vi "liberaToCmd.vi"(5 "set Time":string, 6 "loops":i32=1, 7 "acquire time":u32, 8 "samples":u32=1, 9 "triggered":bool, 10 "decimated":bool, 11 "cmd":T1(ring)=enum."acquireDD") -> (0 "jsonargs":string, 3 "cmd":string)   [LabVIEW 2010]
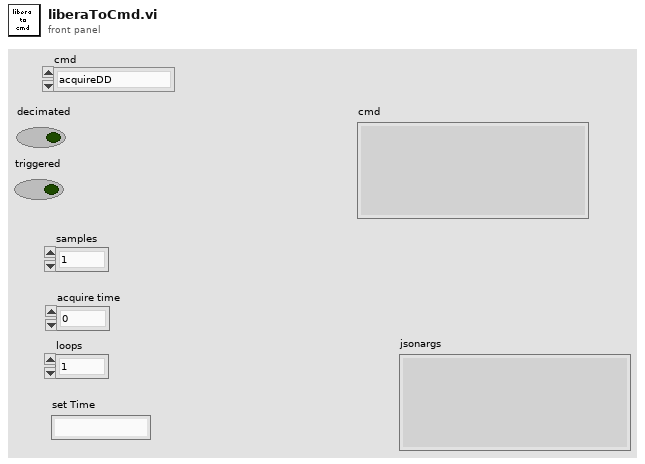
[diagram p1: front panel]
types:
  T1 = enum16{"stopAcquire", "setTime", "acquireAVG", "acquireADCSP", "acquireADCCW", "acquireStream", "acquireDD"}
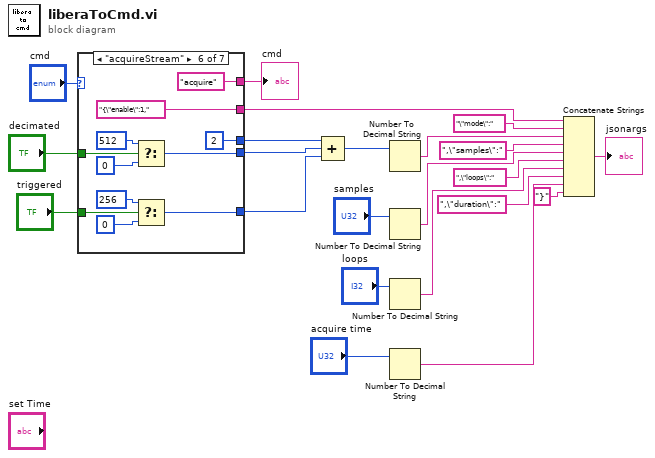
[diagram p0: block diagram]
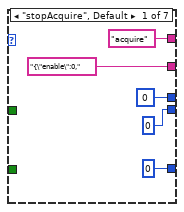
[diagram p2: hidden frame]
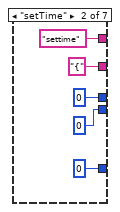
[diagram p3: hidden frame]
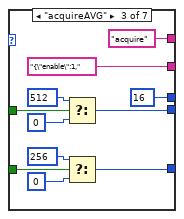
[diagram p4: hidden frame]
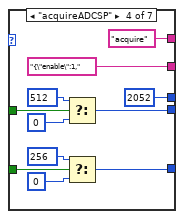
[diagram p5: hidden frame]
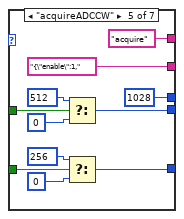
[diagram p6: hidden frame]
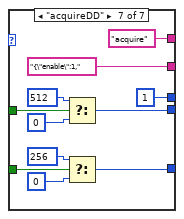
[diagram p7: hidden frame]
diagram:
  n1 = case shown="\"acquireStream\"" "cmd" {
    tunnel: [u32 0 0 u32 16 u32 2052 u32 1028 u32 2 u32 1] -> w21
    tunnel: ["{\"enable\":0," "{" "{\"enable\":1," "{\"enable\":1," "{\"enable\":1," "{\"enable\":1," "{\"enable\":1,"] -> w19
    tunnel: ["acquire" "settime" "acquire" "acquire" "acquire" "acquire" "acquire"] -> w5
    tunnel: [u32 0 ("f") u32 0 ("f") w33 w44 w56 w69 w82] -> w4
    tunnel: [u32 0 ("f") u32 0 ("f") w34 w45 w55 w68 w79] -> w3
    tunnel: "decimated" -> [_ _ w36 w47 w58 w67 w78]
    tunnel: "triggered" -> [_ _ w35 w46 w57 w66 w77]
    frame "stopAcquire", Default {
    }
    frame "setTime" {
    }
    frame "acquireAVG" {
      n2 = Select(t=u32 512, s=w36, f=u32 0) -> (s? t:f=w33:u32)
      n3 = Select(t=u32 256, s=w35, f=u32 0) -> (s? t:f=w34:u32)
    }
    frame "acquireADCSP" {
      n4 = Select(t=u32 512, s=w47, f=u32 0) -> (s? t:f=w44:u32)
      n5 = Select(t=u32 256, s=w46, f=u32 0) -> (s? t:f=w45:u32)
    }
    frame "acquireADCCW" {
      n6 = Select(t=u32 512, s=w58, f=u32 0) -> (s? t:f=w56:u32)
      n7 = Select(t=u32 256, s=w57, f=u32 0) -> (s? t:f=w55:u32)
    }
    frame "acquireStream" {
      n8 = Select(t=u32 512, s=w67, f=u32 0) -> (s? t:f=w69:u32)
      n9 = Select(t=u32 256, s=w66, f=u32 0) -> (s? t:f=w68:u32)
    }
    frame "acquireDD" {
      n10 = Select(t=u32 512, s=w78, f=u32 0) -> (s? t:f=w82:u32)
      n11 = Select(t=u32 256, s=w77, f=u32 0) -> (s? t:f=w79:u32)
    }
  }
  "cmd" <- w5
  n12 = Compound Arithmetic op=ADD(w21, w4, w3) -> (w20:u32)
  n13 = Number To Decimal String(number=w20) -> (decimal integer string=w17:string)  [unwired: 1 in]
  n14 = Number To Decimal String(number="samples") -> (decimal integer string=w14:string)  [unwired: 1 in]
  n15 = Number To Decimal String(number="loops") -> (decimal integer string=w11:string)  [unwired: 1 in]
  n16 = Number To Decimal String(number="acquire time") -> (decimal integer string=w8:string)  [unwired: 1 in]
  n17 = Concatenate Strings(w19, "\"mode\":" ("string"), w17, ",\"samples\":" ("string"), w14, ",\"loops\":" ("string"), w11, ",\"duration\":" ("string"), w8, "}" ("string")) -> (→"jsonargs":string)
